vi "SavingThread.vi"(8 "error in (no error)":errorcluster, 11 "Application Data":T1) -> (0 "error out":errorcluster)   [LabVIEW 2019]
uses:
  Typedefs/#cluster_ApplicationData.ctl
  Typedefs/Acquisition Thread/#cluster_AcqQueueData.ctl
  Typedefs/Acquisition Thread/#enum_AcquisitionTask.ctl
  Typedefs/Saving Thread/#cluster_SavingQueueData.ctl
  Typedefs/Saving Thread/#enum_SavingTask.ctl
  <vilib>/ActorFramework/Message Enqueuer/Message Enqueuer.lvclass
  Typedefs/Saving Thread/#cluster_SavingThreadData.ctl
  Typedefs/Saving Thread/#cluster_SaveData.ctl
  LowLevelError.vi
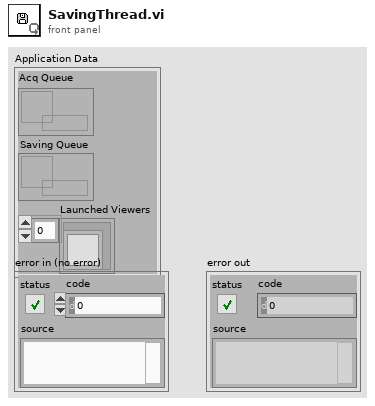
[diagram p1: front panel]
types:
  T1 = typedef "#cluster_ApplicationData.ctl" = cluster{"Acq Queue":refnum<queue>, "Saving Queue":refnum<queue>, "Launched Viewers":refnum<class "Message Enqueuer.lvclass">[]}
  T2 = typedef "#cluster_SavingThreadData.ctl" = cluster{"Measurement Directory":path, "File ref":refnum<k34>, "File opened?":bool}
  T3 = typedef "#cluster_SaveData.ctl" = cluster{"Heart Beat":dbl, "O2":dbl}
  T4 = typedef "#cluster_SavingQueueData.ctl" = cluster{"Task":T5, "Data":variant}
  T5 = typedef "#enum_SavingTask.ctl" = enum16{"Set directory", "Save", "Stop", "Close"}
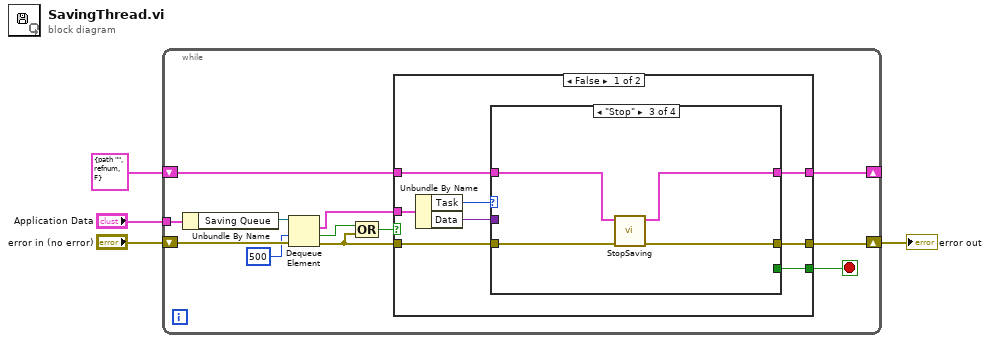
[diagram p0: block diagram]
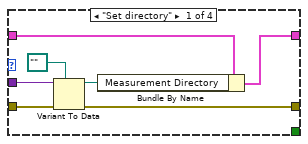
[diagram p2: hidden frame]
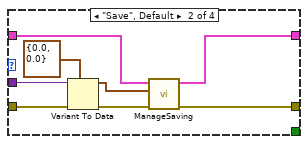
[diagram p3: hidden frame]
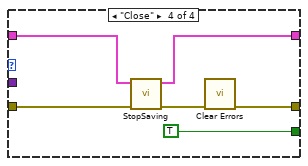
[diagram p4: hidden frame]
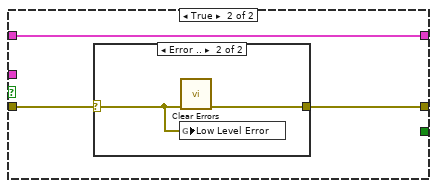
[diagram p5: hidden frame]
diagram:
  n1 = while {
    tunnel: "Application Data" -> [w11]
    shift-right: [w6] -> w2
    shift-left: "error in (no error)" -> [w16]
    shift-right: [w5] -> _
    shift-left: T2 {"Measurement Directory"=path "", "File ref"=refnum, "File opened?"=FALSE} ("Saving Thread Data") -> [w12]
    stop <- w13 stop-if-true
    n2 = Unbundle By Name(w11) -> ("Saving Queue"=w15:refnum<queue>)
    n3 = Dequeue Element(queue=w15, timeout in ms (-1)=500, error in (no error)=w16) -> (element=w14:T4, timed out?=w9:bool, error out=w7:errorcluster)  [unwired: 1 out]
    n4 = Compound Arithmetic op=OR(w9, w7) -> (w8:bool)
    n5 = case shown="False" w8 {
      tunnel: w14 -> [w24 _]
      tunnel: w7 -> [w21 w51]
      tunnel: [w20 _] -> w13
      tunnel: w12 -> [w19 w52]
      tunnel: [w18 w52] -> w5
      tunnel: [w17 w50] -> w6
      frame False {
        n6 = Unbundle By Name(w24) -> ("Task"=w23:T5, "Data"=w22:variant)
        n7 = case shown="\"Stop\"" w23 {
          tunnel: w22 -> [w30 w35 _ _]
          tunnel: w21 -> [w31 w36 w43 w48]
          tunnel: [w25 w38 w40 w46] -> w18
          tunnel: [_ _ _ TRUE] -> w20
          tunnel: w19 -> [w29 w39 w41 w47]
          tunnel: [w28 w37 w42 w44] -> w17
          frame "Set directory" {
            n8 = Variant To Data(error in=w31, type=path "", Variant=w30) -> (data=w26:path, error out=w28:errorcluster)
            n9 = Bundle By Name(cluster=w29, "Measurement Directory"=w26) -> (w25:T2)
          }
          frame "Save", Default {
            n10 = Variant To Data(error in=w36, type=T3 {"Heart Beat"=0.0, "O2"=0.0} ("Save Data"), Variant=w35) -> (data=w32:T3, error out=w33:errorcluster)
            n11 = call "ManageSaving.vi"("error in (no error)"=w33, "Save Data"=w32, "Saving Thread Data in"=w39) -> ("error out"=w37:errorcluster, "Saving Thread Data out"=w38:T2)  [unwired: 7 in]
          }
          frame "Stop" {
            n12 = call "StopSaving.vi"("error in (no error)"=w43, "Saving Thread Data in"=w41) -> ("error out"=w42:errorcluster, "Saving Thread Data out"=w40:T2)  [unwired: 8 in]
          }
          frame "Close" {
            n13 = call "StopSaving.vi"("error in (no error)"=w48, "Saving Thread Data in"=w47) -> ("error out"=w45:errorcluster, "Saving Thread Data out"=w46:T2)  [unwired: 8 in]
            n14 = call <vilib>:"Clear Errors.vi"("error in (no error)"=w45) -> ("error out"=w44:errorcluster)  [unwired: 5 in, 1 out]
          }
        }
      }
      frame True {
        n15 = case shown="Error .." w51 {
          selector: w51 -> [w53 w54]
          tunnel: [w53 w55] -> w50
          frame No Error {
          }
          frame Error {
            n16 = global write "LowLevelError.vi" "Low Level Error"(w54) -> ()
            n17 = call <vilib>:"Clear Errors.vi"("error in (no error)"=w54) -> ("error out"=w55:errorcluster)  [unwired: 5 in, 1 out]
          }
        }
      }
    }
  }
  "error out" <- w2
